vi "Overlay.vi"(8 "error in (no error)":errorcluster, 10 "Image In":T1, 11 "Overlay Base in":refnum<class "Analyze Results Base.lvclass">) -> (0 "error out":errorcluster, 2 "Image out":T1, 3 "Overlay Base out":refnum<class "Analyze Results Base.lvclass">)   [LabVIEW 2020, in "Analyze Results Base.lvclass"]
uses:
  Analyze Results Base.lvclass
  <vilib>/vision/Image Controls.llb/IMAQ Image.ctl
  Analyze Results Base.lvclass/Analyze Results Base.ctl
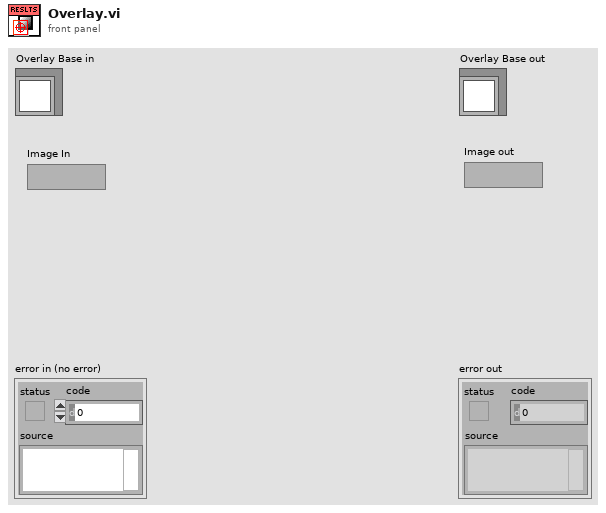
[diagram p1: front panel]
types:
  T1 = typedef "IMAQ Image.ctl" = refnum<image>
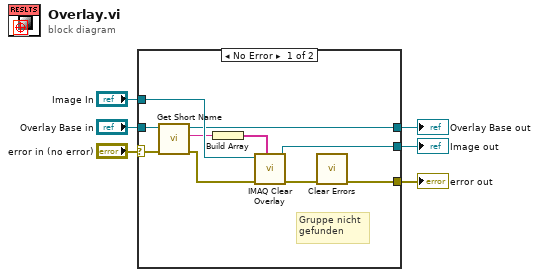
[diagram p0: block diagram]
diagram:
  n1 = case shown="No Error" "error in (no error)" {
    selector: "error in (no error)" -> [w8 w19]
    tunnel: [w12 w19] -> w5
    tunnel: [w10 w18] -> w3
    tunnel: "Overlay Base in" -> [w11 w18]
    tunnel: "Image In" -> [w16 w17]
    tunnel: [w15 w17] -> w1
    frame No Error {
      # "Gruppe nicht\ngefunden"
      n2 = call-dynamic "Get Short Name.vi"("error in (no error)"=w8, "Analyze Results Base in"=w11) -> ("error out"=w7:errorcluster, "Short Name"=w9:string, "Analyze Results Base out"=w10:refnum<class "Analyze Results Base.lvclass">)  [unwired: 7 in]
      n3 = Build Array(w9) -> (w14:string[])
      n4 = call "IMAQ Clear Overlay"("Groups"=w14, "error in (no error)"=w7, "Image"=w16) -> ("error out"=w13:errorcluster, "Image Out"=w15:T1)  [unwired: 7 in]
      n5 = call <vilib>:"Clear Errors.vi"("error in (no error)"=w13) -> ("error out"=w12:errorcluster)  [unwired: 5 in, 1 out]
    }
    frame Error {
    }
  }
  "error out" <- w5
  "Overlay Base out" <- w3
  "Image out" <- w1
